vi "Go To Temperature.vi"(8 "error in (no error)":errorcluster, 9 "Rate (K/s)":dbl=10.0, 10 "Target Temp (K)":dbl=305.0) -> (0 "error out":errorcluster)   [LabVIEW 2016]
uses:
  PPMS Global.vi
  instrument.PPMS2/instrument.PPMS2/instrument.PPMS2.lvclass
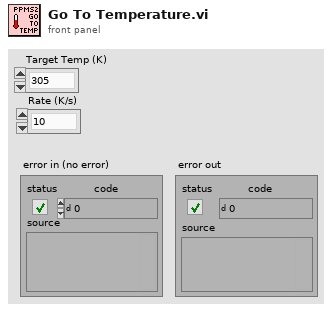
[diagram p1: front panel]
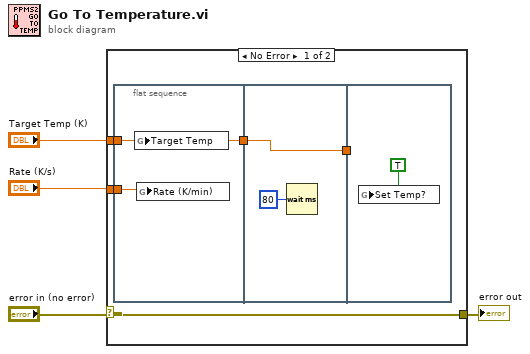
[diagram p0: block diagram]
diagram:
  n1 = case shown="No Error" "error in (no error)" {
    selector: "error in (no error)" -> [w9 w15]
    tunnel: [w9 w15] -> w3
    tunnel: "Rate (K/s)" -> [w8 _]
    tunnel: "Target Temp (K)" -> [w7 _]
    frame No Error {
      n2 = flat-sequence {
        tunnel: w8 -> [w11]
        tunnel: w7 -> [w10]
        tunnel: [w10] -> w6
        tunnel: w6 -> [w12]
        tunnel: [w12] -> w5
        tunnel: w5 -> [_]
        frame #0 {
          n3 = global write "PPMS Global.vi" "Target Temp"(w10) -> ()
          n4 = global write "PPMS Global.vi" "Rate (K/min)"(w11) -> ()
        }
        frame #1 {
          n5 = Wait (ms)(milliseconds to wait=u32 80) -> ()  [unwired: 1 out]
        }
        frame #2 {
          n6 = global write "PPMS Global.vi" "Set Temp?"(TRUE ("Set Field?")) -> ()
        }
      }
    }
    frame Error {
    }
  }
  "error out" <- w3
